vi "AWS_DataFinder_InitResultsList.vi"(11 "Tbl Refnum":refnum<vi>) -> (0 "error out":errorcluster)   [LabVIEW 2014]
doc: "Initialize layout of search results table."
panel:
  # "Initialize layout of search results table."
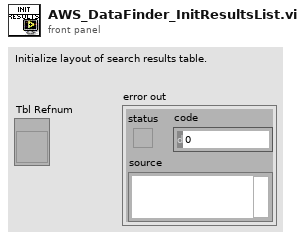
[diagram p1: front panel]
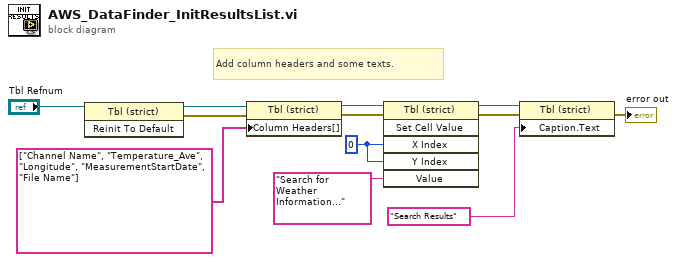
[diagram p0: block diagram]
diagram:
  w7 = u32 0 ("X Index")
  # "Add column headers and some texts."
  n1 = invoke class="Tbl (strict)" method="Reinit To Default"(reference="Tbl Refnum") -> (reference out=w11:refnum<vi>, error out=w1:errorcluster)  [unwired: 2 in, 1 out]
  n2 = property class="Tbl (strict)"(reference=w11, error in=w1, "Column Headers[]"=string[] ["Channel Name", "Temperature_Ave", "Longitude", "MeasurementStartDate", "File Name"] ("Column Header Strings[]")) -> (reference out=w9:refnum<vi>, error out=w8:errorcluster)
  n3 = invoke on="Invoke Node" class="Tbl (strict)" method="Set Cell Value"(reference=w9, error in=w8, "X Index"=w7, "Y Index"=w7, "Value"="Search for Weather  Information...") -> (reference out=w5:refnum<vi>, error out=w4:errorcluster)  [unwired: 1 in, 4 out]
  n4 = property class="Tbl (strict)"(reference=w5, error in=w4, "Caption.Text"="Search Results") -> (error out=→"error out":errorcluster)  [unwired: 1 out]
